vi "ASI Get Start Pos.vi"(9 "piStartY":i32, 10 "piStartX":i32, 11 "iCameraID":i32) -> (1 "piStartY out":i32, 2 "piStartX out":i32, 3 "function return":i32)   [LabVIEW 2012, in "ASICamera2_no_err.lvlib"]
doc: "ASICAMERA_API ASI_ERROR_CODE ASIGetStartPos(int iCameraID, int *piStartX, int *piStartY);"
uses:
  <userlib>/ASICamera2_no_err/ASICamera2_no_err.lvlib
  ASICamera2.dll
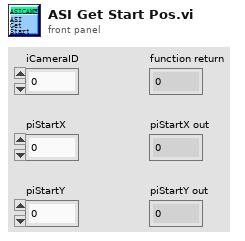
[diagram p1: front panel]
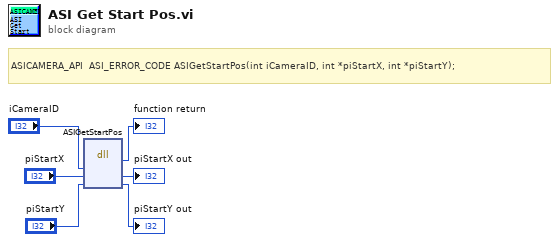
[diagram p0: block diagram]
diagram:
  # "ASICAMERA_API  ASI_ERROR_CODE ASIGetStartPos(int iCameraID, int *piStartX, int *piStartY);"
  n1 = dll-call lib="ASICamera2.*" fn="ASIGetStartPos"("iCameraID"="iCameraID", "piStartX"="piStartX", "piStartY"="piStartY") -> (→"function return":i32, "piStartX"=→"piStartX out":i32, "piStartY"=→"piStartY out":i32)  [unwired: 4 in, 2 out]
